vi "CRYPIC HIDE FRAME.vi"(10 "tFrame":T2) -> (2 "tFrame_Out":T2)   [LabVIEW 2013]
uses:
  <vilib>/Utility/miscctls.llb/LVRectTypeDef.ctl
  CRYStepSetup/CRYStepSetup Global.vi
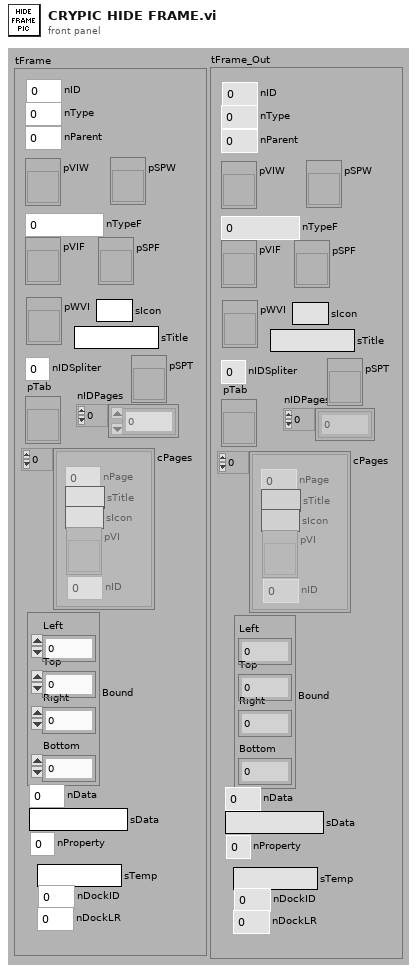
[diagram p1: front panel]
types:
  T1 = typedef "LVRectTypeDef.ctl" = cluster{"Left":i16, "Top":i16, "Right":i16, "Bottom":i16}
  T2 = cluster{"nType":i32, "nParent":i32, "pVIW":refnum<vi>, "pSPW":refnum<vi>, "nTypeF":i32, "pVIF":refnum<vi>, "pSPF":refnum<vi>, "nIDSpliter":i32, "nProperty":i32, "Bound":T1, "nID":i32, "nData":i32, "sData":string, "pWVI":refnum<vi>, "sTitle":string, "cPages":cluster{"nPage":i32, "sTitle":string, "sIcon":string, "pVI":refnum<vi>, "nID":i32}[], "pTab":refnum<vi>, "nIDPages":i32[], "pSPT":refnum<vi>, "sTemp":string, "nDockID":i32, "nDockLR":i32, "sIcon":string}
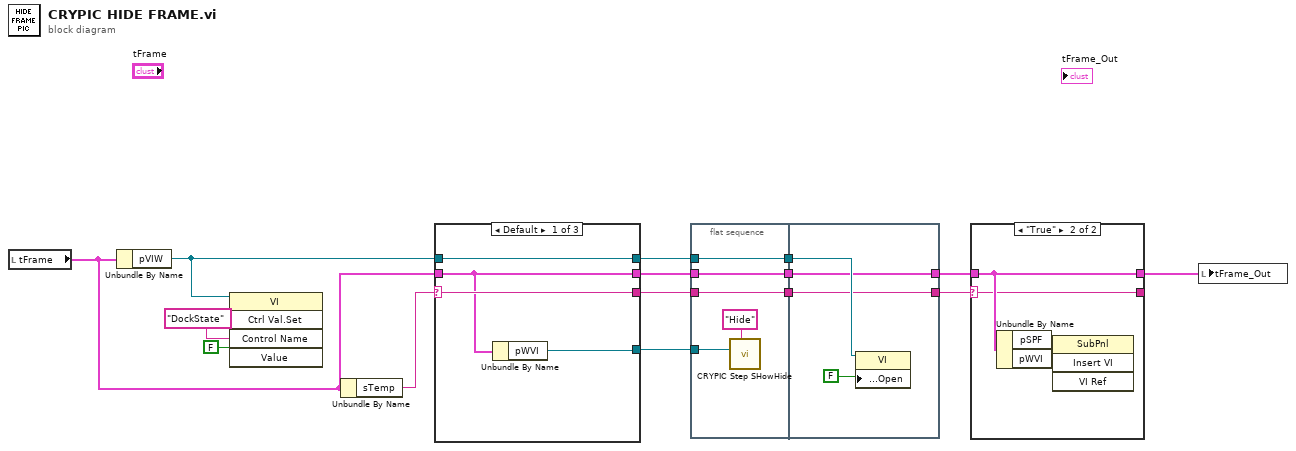
[diagram p0: block diagram]
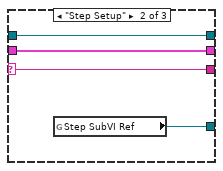
[diagram p3: hidden frame]
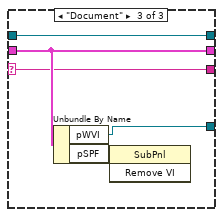
[diagram p4: hidden frame]
diagram:
  n1 = local read "tFrame"() -> (w15:T2)
  n2 = Unbundle By Name(w15) -> ("pVIW"=w11:refnum<vi>)
  n3 = invoke class="VI" method="Ctrl Val.Set"(reference=w11, "Control Name"="DockState", "Value"=FALSE ("bResult")) -> ()  [unwired: 2 in, 5 out]
  n4 = Unbundle By Name(w15) -> ("sTemp"=w5:string)
  n5 = case shown="Default" w5 {
    selector: w5 -> [w18 w21 w26]
    tunnel: w15 -> [w17 w22 w28]
    tunnel: [w17 w22 w28] -> w9
    tunnel: w11 -> [w19 w23 w27]
    tunnel: [w19 w23 w27] -> w10
    tunnel: [w18 w21 w26] -> w8
    tunnel: [w16 w20 w24] -> w1
    frame Default {
      n6 = Unbundle By Name(w17) -> ("pWVI"=w16:refnum<vi>)
    }
    frame "Step Setup" {
      n7 = global read "CRYStepSetup Global.vi" "Step SubVI Ref"() -> (w20:refnum<vi>)
    }
    frame "Document" {
      n8 = Unbundle By Name(w28) -> ("pWVI"=w24:refnum<vi>, "pSPF"=w25:refnum<vi>)
      n9 = invoke class="SubPnl" method="Remove VI"(reference=w25) -> ()  [unwired: 2 in, 3 out]
    }
  }
  n10 = flat-sequence {
    tunnel: w8 -> [w31]
    tunnel: w9 -> [w32]
    tunnel: w10 -> [w33]
    tunnel: [w33] -> w4
    tunnel: [w32] -> w3
    tunnel: [w31] -> w2
    tunnel: w1 -> [w29]
    tunnel: [w35] -> w7
    tunnel: [w34] -> w6
    tunnel: w4 -> [w36]
    tunnel: w3 -> [w35]
    tunnel: w2 -> [w34]
    frame #0 {
      n11 = call "CRYPIC Step SHowHide.vi"("sAction"="Hide", "VIRef"=w29) -> ()  [unwired: 10 in]
    }
    frame #1 {
      n12 = property class="VI"(reference=w36, "Front Panel.Open"=FALSE ("Front Panel Window:Open")) -> ()  [unwired: 1 in, 2 out]
    }
  }
  n13 = case shown="\"True\"" w6 {
    selector: w6 -> [w38 w42]
    tunnel: w7 -> [w39 w43]
    tunnel: [w39 w43] -> w12
    tunnel: [w38 w42] -> _
    frame "False", Default {
    }
    frame "True" {
      n14 = Unbundle By Name(w43) -> ("pSPF"=w41:refnum<vi>, "pWVI"=w40:refnum<vi>)
      n15 = invoke class="SubPnl" method="Insert VI"(reference=w41, "VI Ref"=w40) -> ()  [unwired: 2 in, 4 out]
    }
  }
  n16 = local write "tFrame_Out"(w12) -> ()
